vi "Auto Index_record.vi"(10 "User                   Date                 hr     min      Yields":T2(array[cluster])) -> (2 "Array":T1(array[cluster]))   [LabVIEW 2014, in "Master.lvclass"]
uses:
  Master/Master.lvclass
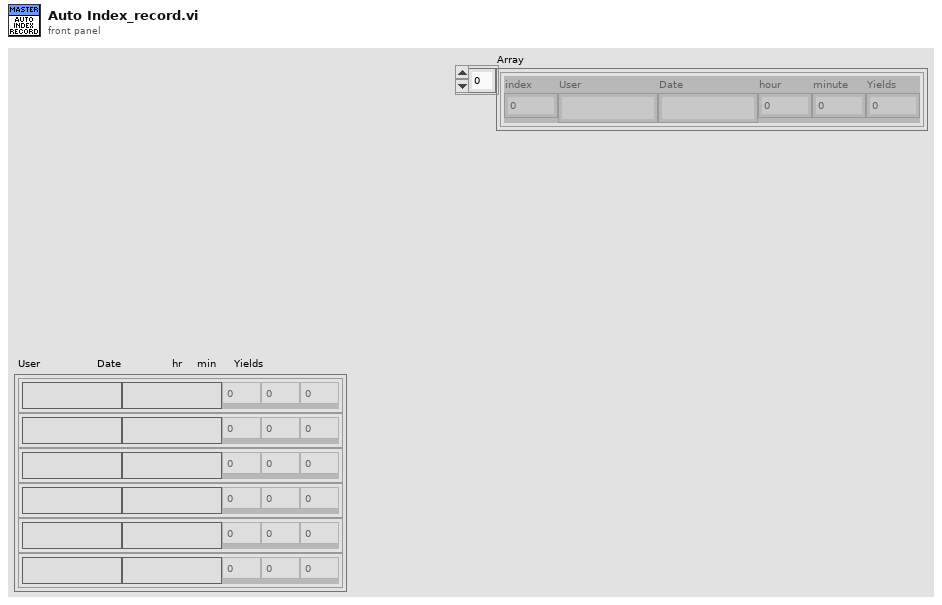
[diagram p1: front panel]
types:
  T1 = cluster{"index":i32, "User":string, "Date":string, "hour":i32, "minute":i32, "Yields":dbl}[]
  T2 = cluster{"User":string, "Date":string, "Yields":dbl, "minute":i32, "hour":i32}[]
  T3 = cluster{"index":i32, "User":string, "Date":string, "minute":i32, "hour":i32, "Yields":dbl}
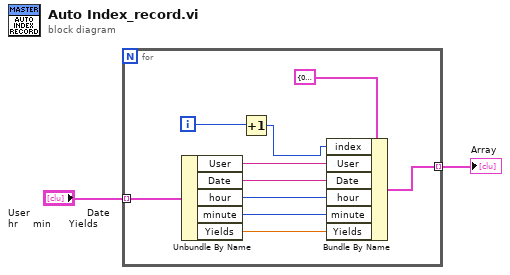
[diagram p0: block diagram]
diagram:
  n1 = for {
    tunnel: "User                   Date                 hr     min      Yields" -> [w12] mode=indexing
    tunnel: [w8] -> w1 mode=indexing
    i -> [w4]
    n2 = Unbundle By Name(w12) -> ("User"=w11:string, "Date"=w10:string, "hour"=w9:i32, "minute"=w6:i32, "Yields"=w5:dbl)
    n3 = Increment(x=w4) -> (x+1=w3:i32)
    n4 = Bundle By Name(cluster=T3 {"index"=0, "User"="", "Date"="", "minute"=0, "hour"=0, "Yields"=0.0}, "index"=w3, "User"=w11, "Date"=w10, "hour"=w9, "minute"=w6, "Yields"=w5) -> (w8:T3)
  }
  "Array" <- w1
